vi "Preferences.vi"(7 "FileList":refnum<vi>, 11 "Files":T1[](array[typedef])) -> (0 "Settings out":T2={"Name of test"="", "Date"=timestamp(0 s since 1904-01-01), "Location"="", "Template"="", "Soundcard"="", "resolution"=32, "Sampling rate"=48000, "Ch1 Gain "=25.0, "Ch2 Gain"=10.0, "Sample time (s)"=0.3, "Pre-trigger (s)"=0.01, "Hammer Threshold"=10.0, "Positions"=12, "Taps/Position"=5, "Set Names"="", "Freq resolution"=10.0, "Hammer cutoff"=0.0, "Mic cutoff"=0.0, "Double bounce "=0.0, "Hammer Cal"=10.0, "dB Offset"=0.0, "Accel Cal"=10.0, "Vibrometer Cal"=0.0, "Mic Cal"=0.0, "Output"=2, "Voltage Cal"=0.01, "Vibrometer Port"="ASRL27::INSTR", "Range"=4, "High Pass"=2, "Bandwidth"=4, "X Range"=[], "Y Range"=[], "dB Spread"=0.0, "Trigger"=0, "Ch_1"=25, "Ch_2"=25, "flip?"=FALSE, "60Hz"=FALSE, "Time offset"=0.0, "Piezo Cal"=1.0, "Default Notes"="", "Tom"=FALSE} {"Ch_2" min=1 step=1; "Ch_1" min=1 max=100 step=1; "Trigger" items=["Hammer (force)", "Self-tap", "Spacebar"]; "Bandwidth" items=["1 kHz"=1, "5 kHz"=5, "10 kHz"=10, "25 kHz"=25, "50 kHz"=50, "100 kHz"=100]; "High Pass" items=["Off", "13 Hz", "104 Hz"]; "Range" items=["10 mm/s"=1, "20 mm/s"=2, "50 mm/s"=5, "100 mm/s"=10, "200 mm/s"=20, "500 mm/s"=50, "1 m/s"=100, "2 m/s"=200]; "Output" items=["Accelerometer", "Speed (from acceleration)", "Microphone", "Vibrometer", "Piezo"]; "Voltage Cal" format="%#_13g"; "Ch2 Gain" format="%#_13g"; "Ch1 Gain" format="%#_13g"; "Double bounce" min=0.0; "Mic cutoff" min=0.0 format="%#_4g"; "Hammer cutoff" min=0.0 format="%#_4g"; "Freq resolution" min=0.0; "Pre-trigger (s)" format="%#_13g"; "Date" format="%<%H:%M\n%d/%m/%y>T"; "resolution" items=["16 bit"=16, "24 bit"=24, "32 bit"=32]; "Sampling rate" items=["22050 samp/s"=22050, "44100 samp/s"=44100, "48000 samp/s"=48000]}, 1 "Success?":bool, 3 "Fixed Files":T1[](array[typedef]))   [LabVIEW 2022 SP3]
uses:
  PreferencesControl.ctl
  Curtin1_Label.ctl
  Mic/Mic_Global.vi
panel:
  out "Cover":bool
  in  "Tab Control":T3(tab)
  in  "CSV?":bool=TRUE
  in  "DAQ":bool
  in  "Vibrometer":bool
  in  "View":bool
  in  "Device":u16(ring) items=["485B39 200083408035100798118210422", "MacBook Pro Microphone", "Microsoft Teams Audio"]
  out "Data Folder:":path=path "/Users/crogers/Desktop/Curtin2/Data"
  in  "Data Folder":bool
  out "Path to preferences":path
  out "Current ScratchPad Settings":string
  in  "Trigger":u16(ring) items=["Hammer (force)", "Self-tap"]
  in  "60Hz?":bool
  in  "F<0?":bool
  in  "Add Color":bool
  in  "Viewing":T4={"Alerts"=FALSE, "Log X Axis"=TRUE, "dB scale"=TRUE, "Averaging"=TRUE, "Fade"=0.8181818181818182, "Centroids?"=TRUE, "line thickness"=1} {"Fade" scale=0.0..1.0}
  in  "Plot Colors":u16(ring) items=["Last Saved", "24 Colors", "rear"]
  in  "Note Files":u16(ring) items=["Default Notes", "Laser Notes", "Original Notes", "Testing Notes"]
  in  "Default Notes":string
  in  "Save As":bool
  in  "remove csv":bool
  in  "Reset":bool
  in  "Type":bool
  in  "Name":string(combo)
  in  "Selection":T5(radio)
  in  "open Folder":bool
  in  "Cancel Button":bool
  in  "OK Button":bool
  out "Version":string
  # "Hz"
  # "dB"
  # "dB"
  # "sec"
  # "sec"
  # "mV/Pa"
  # "mV/m/s2"
  # "mV/mm/s"
  # "V/N"
  # "sec"
  # "sec"
  # "mV/N"
  # "a.u."
  # "a.u."
  # "sec"
  # "not visible"
  # "no fade"
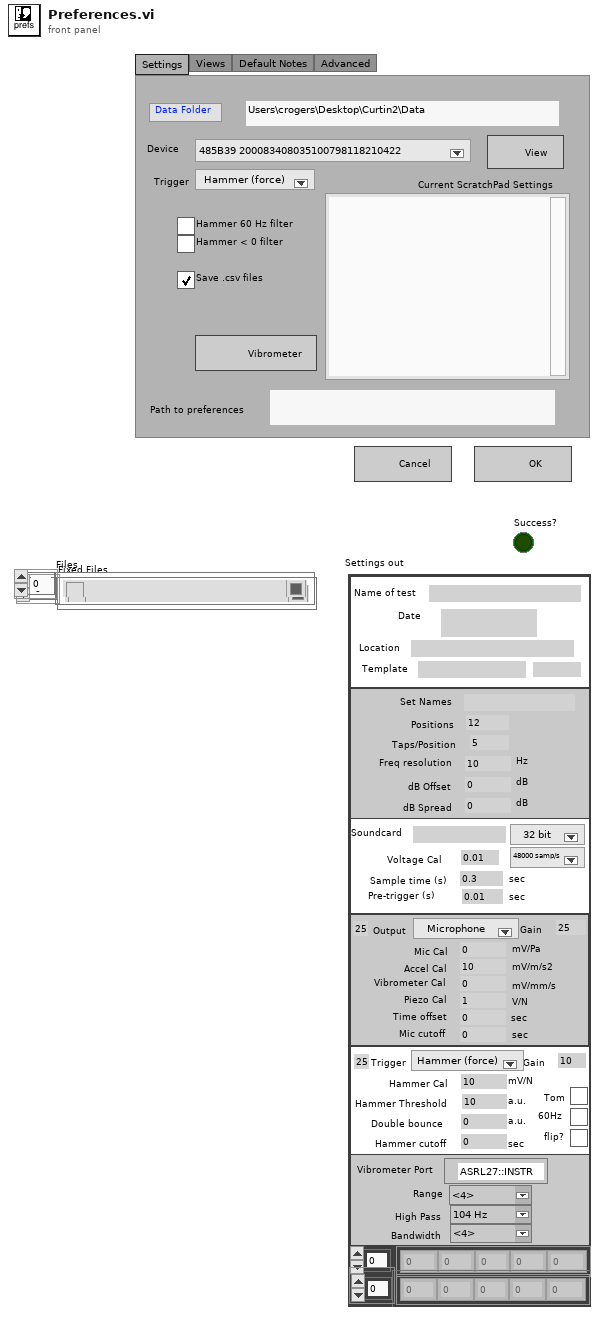
[diagram p1: front panel]
types:
  T1 = typedef "Curtin1_Label.ctl" = cluster{"Show?":bool, "Name":string, "Color":u32, "Path":path, "Show Notes":bool}
  T2 = typedef "PreferencesControl.ctl" = cluster{"Name of test":string, "Date":timestamp, "Location":string, "Template":string, "Soundcard":string, "resolution":u16, "Sampling rate":u16, "Ch1 Gain ":dbl, "Ch2 Gain":dbl, "Sample time (s)":dbl, "Pre-trigger (s)":dbl, "Hammer Threshold":dbl, "Positions":i16, "Taps/Position":i16, "Set Names":string, "Freq resolution":dbl, "Hammer cutoff":dbl, "Mic cutoff":dbl, "Double bounce ":dbl, "Hammer Cal":dbl, "dB Offset":dbl, "Accel Cal":dbl, "Vibrometer Cal":dbl, "Mic Cal":dbl, "Output":u16, "Voltage Cal":dbl, "Vibrometer Port":refnum<visa-resource-name>, "Range":u16, "High Pass":u16, "Bandwidth":u16, "X Range":cluster{"Minimum":dbl, "Maximum":dbl, "Increment":dbl, "Minor Increment":dbl, "Start":dbl}[], "Y Range":cluster{"Minimum":dbl, "Maximum":dbl, "Increment":dbl, "Minor Increment":dbl, "Start":dbl}[], "dB Spread":dbl, "Trigger":u16, "Ch_1":u8, "Ch_2":u8, "flip?":bool, "60Hz":bool, "Time offset":dbl, "Piezo Cal":dbl, "Default Notes":string, "Tom":bool}
  T3 = enum32{"Settings", "Views", "Default Notes", "Advanced"}
  T4 = cluster{"Alerts":bool, "Log X Axis":bool, "dB scale":bool, "Averaging":bool, "Fade":dbl, "Centroids?":bool, "line thickness":u8}
  T5 = enum32{"No Selection", "Rename", "Recalculate", "Export", "Delete", "Duplicate"}
  T6 = enum32{"Invalid", "Default", "Floating", "Floating/Auto-Hide", "Modal"}
  T7 = enum16{"big-endian, network order", "native, host order", "little-endian"}
  T8 = enum32{"No Selection", "Rename", "Recalculate", "Export", "Delete"}
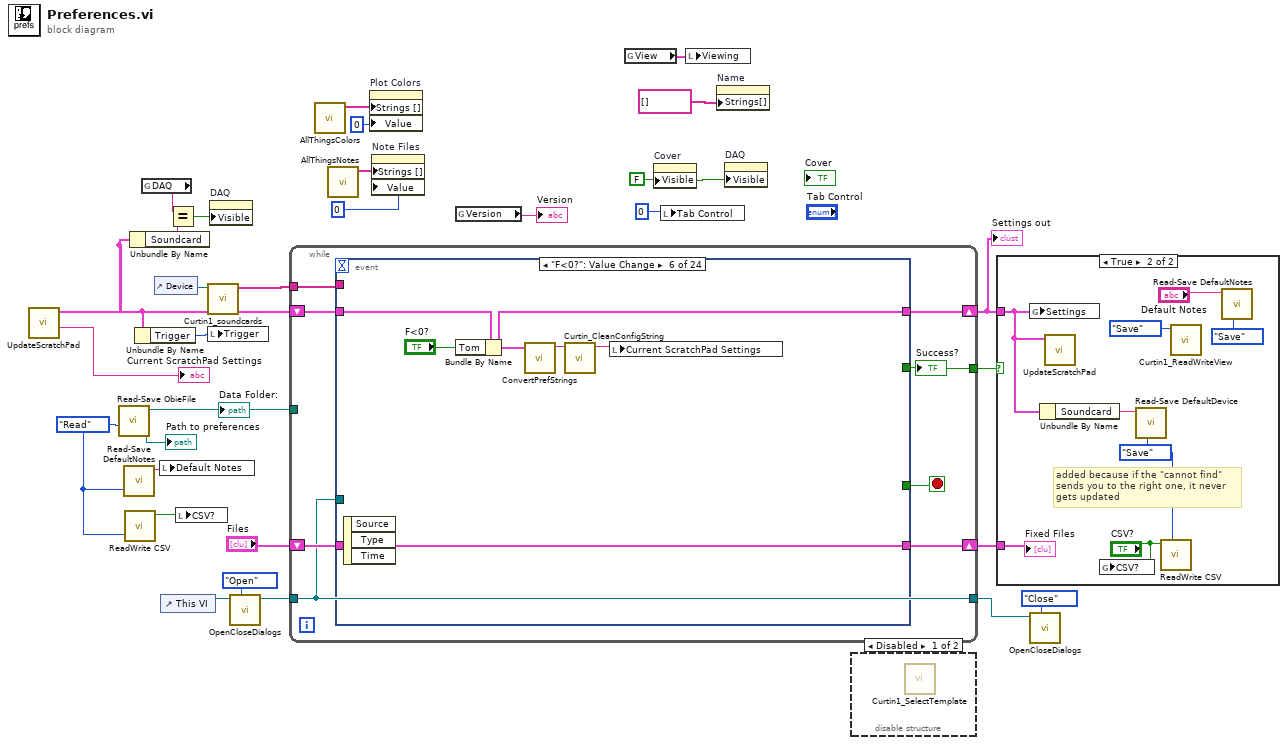
[diagram p0: block diagram]
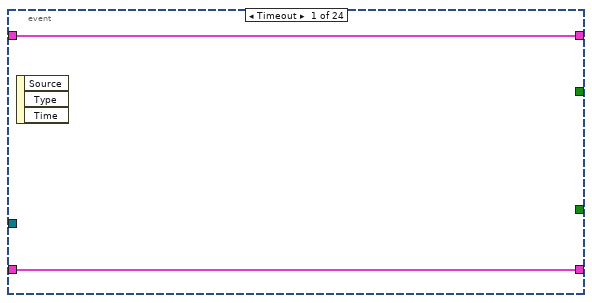
[diagram p4: hidden frame]
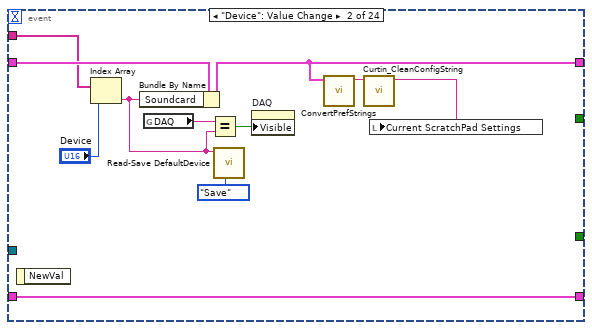
[diagram p5: hidden frame]
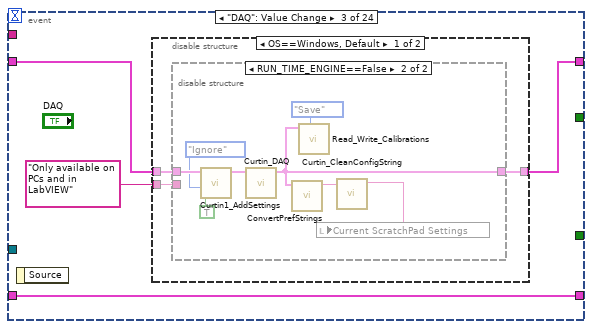
[diagram p6: hidden frame]
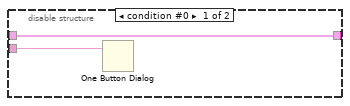
[diagram p7: hidden frame]
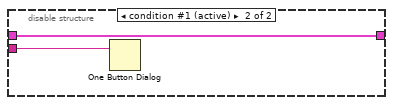
[diagram p8: hidden frame]
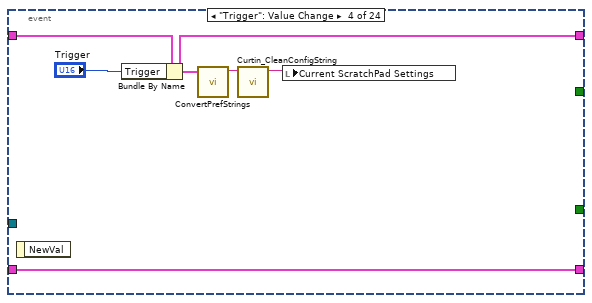
[diagram p9: hidden frame]
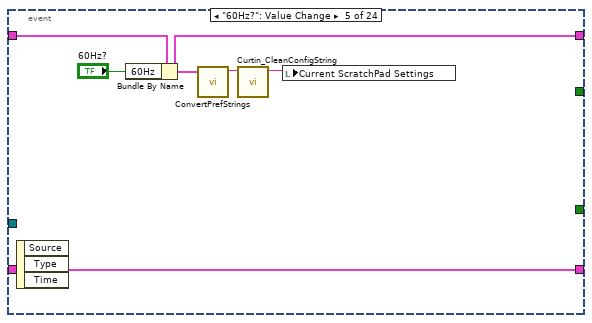
[diagram p10: hidden frame]
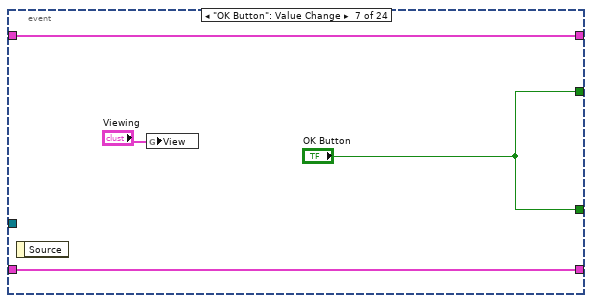
[diagram p11: hidden frame]
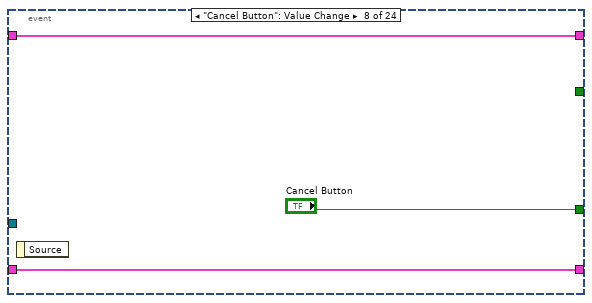
[diagram p12: hidden frame]
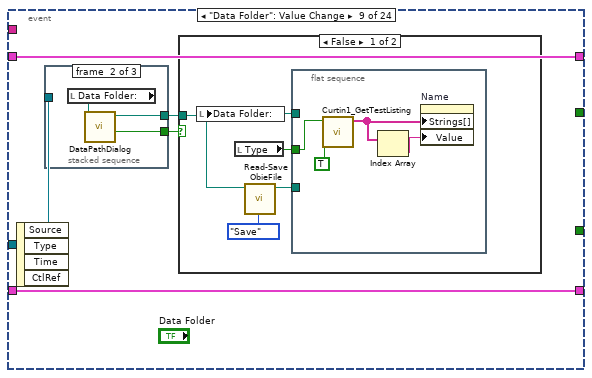
[diagram p13: hidden frame]
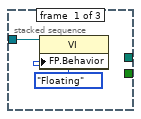
[diagram p14: hidden frame]
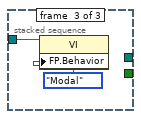
[diagram p15: hidden frame]
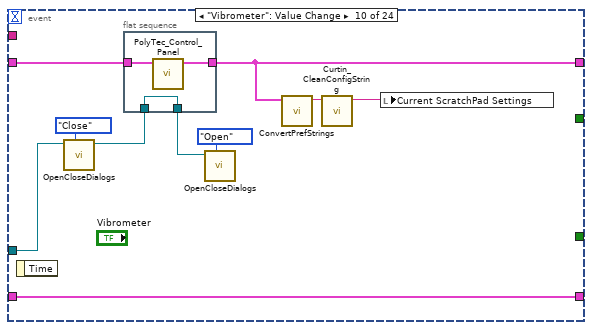
[diagram p17: hidden frame]
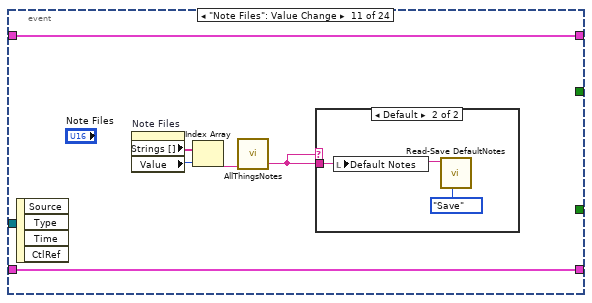
[diagram p18: hidden frame]
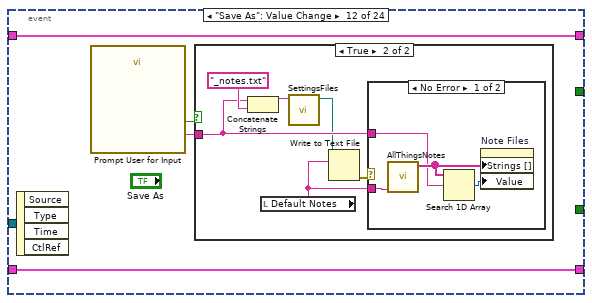
[diagram p20: hidden frame]
diagram:
  w10 = FALSE ("Visible")
  w2 = enum16{"Save", "Read"}."Read" ("Task")
  n1 = call "UpdateScratchPad.vi"() -> ("Settings"=→"Current ScratchPad Settings":string, "Settings Out"=w9:T2)  [unwired: 10 in]
  n2 = call "Read-Save ObieFile.vi"("Task"=w2) -> ("Pref Path"=→"Path to preferences":path, "DataPath Out"=w25:path)  [unwired: 8 in, 1 out]
  "Data Folder:" <- w25
  n3 = call "Read-Save DefaultNotes.vi"("Task"=w2) -> ("Notes Out"=w29:string)  [unwired: 9 in, 1 out]
  n4 = call "ReadWrite CSV.vi"("Task"=w2) -> ("csv Out"=w1:bool)  [unwired: 10 in]
  n5 = Unbundle By Name(w9) -> ("Soundcard"=w12:string)
  n6 = Unbundle By Name(w9) -> ("Trigger"=w20:u16)
  n7 = global read "Mic_Global.vi" "DAQ"() -> (w11:string)
  n8 = control-ref of="Device"() -> (w24:refnum<vi>)
  n9 = local write "Default Notes"(w29) -> ()
  n10 = control-ref of="This VI"() -> (w6:refnum<vi>)
  n11 = Equal?(x=w11, y=w12) -> (x = y?=w13:bool)
  n12 = local write "CSV?"(w1) -> ()
  n13 = call "Curtin1_soundcards.vi"("Settings In"=w9, "device:"=w24) -> ("Settings Out"=w19:T2, "Devices"=w26:string[])  [unwired: 8 in]
  n14 = local write "Trigger"(w20) -> ()
  n15 = property on="DAQ" class="Bool"("Visible"=w13) -> ()  [unwired: 2 in, 2 out]
  n16 = call "OpenCloseDialogs.vi"("Task"=enum16{"Open", "Close"}."Open", "VI in"=w6) -> ("VI out"=w3:refnum<vi>)  [unwired: 8 in, 1 out]
  n17 = while {
    tunnel: w26 -> [w39]
    shift-right: [w37] -> w30
    shift-left: w19 -> [w38]
    tunnel: [w36] -> w28
    tunnel: w25 -> [_]
    shift-right: [w35] -> w16
    shift-left: "Files" -> [w34]
    tunnel: [w33] -> w4
    tunnel: w3 -> [w33]
    stop <- w40 stop-if-true
    n18 = event shown="[5] \"F<0?\": Value Change" {
      selector: _ -> [_ _ _ _ _ _ _ _ _ _ _ _ _ _ _ _ _ _ _ _ _ _ _ _]
      dyn-events: _ -> [_ _ _ _ _ _ _ _ _ _ _ _ _ _ _ _ _ _ _ _ _ _ _ _]
      timeout: _ -> [_ _ _ _ _ _ _ _ _ _ _ _ _ _ _ _ _ _ _ _ _ _ _ _]
      tunnel: [_ _ _ _ _ _ "OK Button" "Cancel Button" _ _ _ _ _ _ _ _ _ _ _ _ _ _ _ w252] -> w40
      tunnel: w39 -> [_ w51 _ _ _ _ _ _ _ _ _ _ _ _ _ _ _ _ _ _ _ _ _ _]
      tunnel: [_ _ _ _ _ _ "OK Button" _ _ _ _ _ _ _ _ _ _ _ _ _ _ _ _ _] -> w36
      tunnel: w38 -> [w42 w52 w54 w78 w84 w90 w93 w96 w102 w126 w136 w142 w154 w161 w172 w177 w187 w193 w195 w204 w218 w228 w248 w251]
      tunnel: [w42 w44 w55 w74 w81 w87 w93 w96 w102 w124 w136 w142 w154 w161 w172 w177 w187 w193 w195 w202 w218 w228 w248 w251] -> w37
      tunnel: [w41 w50 w57 w76 w83 w89 w91 w95 w100 w127 w131 w139 w153 w155 w171 w176 w185 w192 w194 w203 w217 w227 w249 w250] -> w35
      tunnel: w34 -> [w41 w50 w57 w76 w83 w89 w91 w95 w100 w127 w131 w139 w153 w155 w171 w176 w185 w192 w194 w203 _ w227 w249 w250]
      tunnel: w33 -> [_ _ _ _ _ _ _ _ w98 w121 _ _ _ _ _ _ _ _ _ w200 _ w224 _ _]
      event Timeout {
        n19 = event-data() -> ()  [unwired: 1 in, 3 out]
      }
      event "Device": Value Change {
        n20 = event-data() -> ()  [unwired: 1 in, 1 out]
        n21 = Index Array(array=w51, index="Device") -> (element=w46:string)
        n22 = Bundle By Name(cluster=w52, "Soundcard"=w46) -> (w44:T2)
        n23 = global read "Mic_Global.vi" "DAQ"() -> (w48:string)
        n24 = Equal?(x=w48, y=w46) -> (x = y?=w47:bool)
        n25 = call "Read-Save DefaultDevice.vi"("Task"=enum16{"Save", "Read"}."Save", "Soundcard"=w46) -> ()  [unwired: 8 in, 2 out]
        n26 = property on="DAQ" class="Bool"("Visible"=w47) -> ()  [unwired: 2 in, 2 out]
        n27 = call "ConvertPrefStrings.vi"("Settings"=w44) -> ("String Out"=w45:string)  [unwired: 9 in, 1 out]
        n28 = call "Curtin_CleanConfigString.vi"("String in"=w45) -> ("String out"=w43:string)  [unwired: 10 in]
        n29 = local write "Current ScratchPad Settings"(w43) -> ()
      }
      event "DAQ": Value Change {
        n30 = event-data() -> ()  [unwired: 1 in, 1 out]
        n31 = disable-structure shown="OS==Windows, Default" {
          disable-tunnel: "Only available on PCs and in LabVIEW" ("message") -> [w60 w72]
          disable-tunnel: w54 -> [w59 w71]
          disable-tunnel: [w58 w71] -> w55
          frame condition #0 {
            n32 = disable-structure shown="RUN_TIME_ENGINE==False" {
              disable-tunnel: w60 -> [w62 _]
              disable-tunnel: w59 -> [w61 w70]
              disable-tunnel: [w61 w68] -> w58
              frame condition #0 {
                n33 = One Button Dialog(message=w62) -> ()  [unwired: 1 in, 1 out]
              }
              frame condition #1 (active) {
                n34 = call "Curtin1_AddSettings.vi"("Date?"=TRUE, "Check?"=enum16{"Ignore", "Check", "Replace"}."Ignore", "Settings in"=w70) -> ("Settings Out"=w69:T2)  [unwired: 7 in, 1 out]
                n35 = call "Curtin_DAQ.vi"("Settings"=w69) -> ("Settings out"=w68:T2)  [unwired: 10 in]
                n36 = call "ConvertPrefStrings.vi"("Settings"=w68) -> ("String Out"=w66:string)  [unwired: 9 in, 1 out]
                n37 = call "Read_Write_Calibrations.vi"("Task"=enum16{"Save", "Read", "List"}."Save", "Settings in"=w68) -> ()  [unwired: 7 in, 3 out]
                n38 = call "Curtin_CleanConfigString.vi"("String in"=w66) -> ("String out"=w65:string)  [unwired: 10 in]
                n39 = local write "Current ScratchPad Settings"(w65) -> ()
              }
            }
          }
          frame condition #1 (active) {
            n40 = One Button Dialog(message=w72) -> ()  [unwired: 1 in, 1 out]
          }
        }
      }
      event "Trigger": Value Change {
        n41 = event-data() -> ()  [unwired: 1 in, 1 out]
        n42 = Bundle By Name(cluster=w78, "Trigger"="Trigger") -> (w74:T2)
        n43 = call "ConvertPrefStrings.vi"("Settings"=w74) -> ("String Out"=w75:string)  [unwired: 9 in, 1 out]
        n44 = call "Curtin_CleanConfigString.vi"("String in"=w75) -> ("String out"=w73:string)  [unwired: 10 in]
        n45 = local write "Current ScratchPad Settings"(w73) -> ()
      }
      event "60Hz?": Value Change {
        n46 = event-data() -> ()  [unwired: 1 in, 3 out]
        n47 = Bundle By Name(cluster=w84, "60Hz"="60Hz?") -> (w81:T2)
        n48 = call "ConvertPrefStrings.vi"("Settings"=w81) -> ("String Out"=w82:string)  [unwired: 9 in, 1 out]
        n49 = call "Curtin_CleanConfigString.vi"("String in"=w82) -> ("String out"=w80:string)  [unwired: 10 in]
        n50 = local write "Current ScratchPad Settings"(w80) -> ()
      }
      event "F<0?": Value Change {
        n51 = event-data() -> ()  [unwired: 1 in, 3 out]
        n52 = Bundle By Name(cluster=w90, "Tom"="F<0?") -> (w87:T2)
        n53 = call "ConvertPrefStrings.vi"("Settings"=w87) -> ("String Out"=w88:string)  [unwired: 9 in, 1 out]
        n54 = call "Curtin_CleanConfigString.vi"("String in"=w88) -> ("String out"=w86:string)  [unwired: 10 in]
        n55 = local write "Current ScratchPad Settings"(w86) -> ()
      }
      event "OK Button": Value Change {
        n56 = event-data() -> ()  [unwired: 1 in, 1 out]
        n57 = global write "Mic_Global.vi" "View"("Viewing") -> ()
      }
      event "Cancel Button": Value Change {
        n58 = event-data() -> ()  [unwired: 1 in, 1 out]
      }
      event "Data Folder": Value Change {
        n59 = event-data() -> ()  [unwired: 1 in, 4 out]
        n60 = stacked-sequence {
          tunnel: [_ w106 _] -> w101
          tunnel: [_ w105 _] -> w99
          tunnel: w98 -> [w104 _ w109]
          frame #0 {
            n61 = property class="VI"(reference=w104, "FP.Behavior"=T6."Floating" ("Front Panel Window:Behavior")) -> ()  [unwired: 1 in, 2 out]
          }
          frame #1 {
            n62 = local read "Data Folder:"() -> (w107:path)
            n63 = call "DataPathDialog.vi"("Path"=w107) -> ("canceled?"=w105:bool, "Path out"=w106:path)  [unwired: 9 in]
          }
          frame #2 {
            n64 = property class="VI"(reference=w109, "FP.Behavior"=T6."Modal" ("Front Panel Window:Behavior")) -> ()  [unwired: 1 in, 2 out]
          }
        }
        n65 = case shown="False" w99 {
          tunnel: w101 -> [w111 _]
          frame False {
            n66 = local write "Data Folder:"(w111) -> ()
            n67 = local read "Type"() -> (w113:bool)
            n68 = call "Read-Save ObieFile.vi"("Task"=enum16{"Save", "Read"}."Save", "DataPath"=w111) -> ("DataPath Out"=w110:path)  [unwired: 7 in, 2 out]
            n69 = flat-sequence {
              tunnel: w111 -> [_]
              tunnel: w113 -> [w115]
              tunnel: w110 -> [_]
              frame #0 {
                n70 = call "Curtin1_GetTestListing.vi"("Rebuild"=TRUE, "Type"=w115) -> ("Array"=w117:string[])  [unwired: 9 in]
                n71 = Index Array(array=w117) -> (element=w116:string)  [unwired: 1 in]
                n72 = property on="Name" class="CmbBox"("Strings[]"=w117, "Value"=w116) -> ()  [unwired: 2 in, 2 out]
              }
            }
          }
          frame True {
          }
        }
      }
      event "Vibrometer": Value Change {
        n73 = event-data() -> ()  [unwired: 1 in, 1 out]
        n74 = call "OpenCloseDialogs.vi"("Task"=enum16{"Open", "Close"}."Close", "VI in"=w121) -> ("VI out"=w119:refnum<vi>)  [unwired: 8 in, 1 out]
        n75 = flat-sequence {
          tunnel: w126 -> [w130]
          tunnel: [w129] -> w124
          tunnel: [w128] -> w120
          tunnel: w119 -> [w128]
          frame #0 {
            n76 = call "PolyTec_Control_Panel.vi"("Settings in"=w130) -> ("Settings Out"=w129:T2)  [unwired: 8 in, 2 out]
          }
        }
        n77 = call "OpenCloseDialogs.vi"("Task"=enum16{"Open", "Close"}."Open", "VI in"=w120) -> ()  [unwired: 8 in, 2 out]
        n78 = call "ConvertPrefStrings.vi"("Settings"=w124) -> ("String Out"=w125:string)  [unwired: 9 in, 1 out]
        n79 = call "Curtin_CleanConfigString.vi"("String in"=w125) -> ("String out"=w123:string)  [unwired: 10 in]
        n80 = local write "Current ScratchPad Settings"(w123) -> ()
      }
      event "Note Files": Value Change {
        n81 = event-data() -> ()  [unwired: 1 in, 4 out]
        n82 = property on="Note Files" class="Ring (strict)"() -> ("Strings []"=w135:string[], "Value"=w133:u16)  [unwired: 2 in, 2 out]
        n83 = Index Array(array=w135, index=w133) -> (element=w134:string)
        n84 = call "AllThingsNotes.vi"("Choice"=w134) -> ("Text"=w132:string)  [unwired: 9 in, 1 out]
        n85 = case shown="Default" w132 {
          tunnel: w132 -> [_ w137]
          frame "" {
          }
          frame Default {
            n86 = local write "Default Notes"(w137) -> ()
            n87 = call "Read-Save DefaultNotes.vi"("Task"=enum16{"Save", "Read"}."Save", "Notes"=w137) -> ()  [unwired: 8 in, 2 out]
          }
        }
      }
      event "Save As": Value Change {
        n88 = event-data() -> ()  [unwired: 1 in, 4 out]
        n89 = call "Prompt User for Input"() -> ("Filename"=w140:string, "OK"=w141:bool)  [unwired: 17 in, 1 out]
        n90 = case shown="True" w141 {
          tunnel: w140 -> [_ w146]
          frame False {
          }
          frame True {
            n91 = Concatenate Strings(w146, "_notes.txt" ("pattern")) -> (w145:string)
            n92 = local read "Default Notes"() -> (w147:string)
            n93 = call "SettingsFiles.vi"("settings file name"=w145) -> ("file path"=w144:path)  [unwired: 9 in, 1 out]
            n94 = Write to Text File(file (use dialog)=w144, text=w147) -> (error out=w143:errorcluster)  [unwired: 2 in, 2 out]
            n95 = case shown="No Error" w143 {
              tunnel: w147 -> [w152 _]
              tunnel: w146 -> [w149 _]
              frame No Error {
                n96 = call "AllThingsNotes.vi"("Choice"=w152) -> ("Array"=w150:string[])  [unwired: 9 in, 1 out]
                n97 = Search 1D Array(1D array=w150, element=w149) -> (index of element=w151:i32)  [unwired: 1 in]
                n98 = property on="Note Files" class="Ring (strict)"("Strings []"=w150, "Value"=w151) -> ()  [unwired: 2 in, 2 out]
              }
              frame Error {
              }
            }
          }
        }
      }
      event "Default Notes": Value Change {
        n99 = event-data() -> ()  [unwired: 1 in, 4 out]
      }
      event "Selection": Value Change {
        n100 = event-data() -> ()  [unwired: 1 in, 2 out]
        n101 = local read "Type"() -> (w156:bool)
        n102 = call "Curtin1_AdvancedPrefs.vi"("Type"=w156, "Selection"="Selection", "Instrument:Test Name"="Name") -> ("Selection out"=w158:T8, "message"=w157:string)  [unwired: 7 in]
        n103 = local write "Selection"(w158) -> ()
        n104 = case shown="Default" w157 {
          selector: w157 -> [_ w166]
          tunnel: w156 -> [_ w163]
          frame "" {
          }
          frame Default {
            n105 = One Button Dialog(message=w166) -> ()  [unwired: 1 in, 1 out]
            n106 = call "Curtin1_GetTestListing.vi"("Rebuild"=TRUE, "Type"=w163) -> ("Array"=w165:string[])  [unwired: 9 in]
            n107 = Index Array(array=w165) -> (element=w164:string)  [unwired: 1 in]
            n108 = property on="Name" class="CmbBox"("Strings[]"=w165, "Value"=w164) -> ()  [unwired: 2 in, 2 out]
          }
        }
      }
      event "Type": Value Change {
        n109 = event-data() -> ()  [unwired: 1 in, 2 out]
        n110 = property on="Cover" class="Bool (strict)"("Visible"=TRUE) -> ()  [unwired: 2 in, 2 out]
        n111 = call "Curtin1_GetTestListing.vi"("Rebuild"=FALSE, "Type"="Type") -> ("Array"=w175:string[])  [unwired: 9 in]
        n112 = Index Array(array=w175) -> (element=w174:string)  [unwired: 1 in]
        n113 = property on="Name" class="CmbBox"("Strings[]"=w175, "Value"=w174) -> (error out=w168:errorcluster)  [unwired: 2 in, 1 out]
        n114 = property on="Cover" class="Bool (strict)"(error in=w168, "Visible"=FALSE) -> ()  [unwired: 1 in, 2 out]
      }
      event "Tab Control": Value Change {
        n115 = event-data() -> ("NewVal"=w178:T3)  [unwired: 1 in]
        n116 = case shown="\"Advanced\"" w178 {
          frame "Settings", Default {
          }
          frame "Advanced" {
            n117 = property on="Name" class="CmbBox"() -> ("Strings[]"=w181:string[])  [unwired: 2 in, 2 out]
            n118 = Array Size(array=w181) -> (size(s)=w180:i32)
            n119 = case shown="0" w180 {
              tunnel: string[] ["Loading..."] ("Strings []") -> [_ w182]
              frame Default {
              }
              frame 0 {
                # "First Run"
                n120 = property on="Type" class="Bool (strict)"("Val(Sgnl)"=FALSE ("Value (Signaling)")) -> ()  [unwired: 2 in, 2 out]
                n121 = property on="Name" class="CmbBox"("Strings[]"=w182) -> ()  [unwired: 2 in, 2 out]
              }
            }
          }
        }
      }
      event "Reset": Value Change {
        n122 = event-data() -> ()  [unwired: 1 in, 1 out]
        n123 = call "Curtin1_GlobalFolder.vi"() -> ("LabVIEW Data Path"=w184:path)  [unwired: 1 in, 1 out]
        n124 = call "DefaultSettings.vi"("Task"=enum16{"Load to VI", "Save to Disk"}."Save to Disk", "path (use dialog)"=w184) -> ("No Errors?"=w186:bool)  [unwired: 9 in]
        n125 = case shown="False" w186 {
          frame False {
            n126 = One Button Dialog(message="Error in saving files") -> ()  [unwired: 1 in, 1 out]
          }
          frame True {
            n127 = One Button Dialog(message="Success") -> ()  [unwired: 1 in, 1 out]
          }
        }
      }
      event "open Folder": Value Change {
        n128 = event-data() -> ()  [unwired: 1 in, 1 out]
        n129 = call "Curtin1_GlobalFolder.vi"() -> ("LabVIEW Data Path"=w191:path)  [unwired: 1 in, 1 out]
        n130 = call "OpenFolder.vi"("LabVIEW Data Path"=w191) -> ()  [unwired: 11 in]
      }
      event "Name": Value Change {
        n131 = event-data() -> ()  [unwired: 1 in, 4 out]
      }
      event "View": Value Change {
        n132 = event-data() -> ()  [unwired: 1 in, 1 out]
        n133 = call "OpenCloseDialogs.vi"("Task"=enum16{"Open", "Close"}."Close", "VI in"=w200) -> ("error out"=w197:errorcluster, "VI out"=w196:refnum<vi>)  [unwired: 8 in]
        n134 = case shown="True" "View" {
          tunnel: w204 -> [w207 w214]
          tunnel: [w207 w209] -> w202
          tunnel: [w206 w208] -> w198
          tunnel: w197 -> [w206 w208]
          frame False {
          }
          frame True {
            n135 = call "Curtin1_AddSettings.vi"("Date?"=TRUE, "Check?"=enum16{"Ignore", "Check", "Replace"}."Ignore", "Settings in"=w214) -> ("Settings Out"=w215:T2)  [unwired: 7 in, 1 out]
            n136 = call "Curtin1_ViewMics.vi"("Settings"=w215) -> ("Settings Out"=w209:T2)  [unwired: 10 in]
            n137 = call "ConvertPrefStrings.vi"("Settings"=w209) -> ("String Out"=w213:string)  [unwired: 9 in, 1 out]
            n138 = call "Curtin_CleanConfigString.vi"("String in"=w213) -> ("String out"=w212:string)  [unwired: 10 in]
            n139 = local write "Current ScratchPad Settings"(w212) -> ()
          }
        }
        n140 = call "OpenCloseDialogs.vi"("Task"=enum16{"Open", "Close"}."Open", "error in (no error)"=w198, "VI in"=w196) -> ()  [unwired: 7 in, 2 out]
      }
      event "Plot Colors": Value Change {
        n141 = event-data() -> ()  [unwired: 1 in, 1 out]
        n142 = flat-sequence {
          tunnel: "FileList" -> [w223]
          tunnel: [w222] -> w217
          frame #0 {
            # "load into CurrentColors"
            n143 = property on="Plot Colors" class="Ring (strict)"() -> ("Strings []"=w220:string[], "Value"=w221:u16)  [unwired: 2 in, 2 out]
            n144 = Index Array(array=w220, index=w221) -> (element=w219:string)
            n145 = call "AllThingsColors.vi"("Choice"=w219) -> ()  [unwired: 10 in, 1 out]
          }
          frame #1 {
            # "replot"
            n146 = call "Recolor.vi"("Array in"=w223) -> ("Files"=w222:T1[])  [unwired: 10 in]
          }
        }
      }
      event "Add Color": Value Change {
        n147 = event-data() -> ()  [unwired: 1 in, 1 out]
        n148 = stacked-sequence {
          tunnel: [_ w232 _] -> w226
          tunnel: [_ w231 _] -> w225
          tunnel: w224 -> [w229 _ w233]
          frame #0 {
            n149 = property class="VI"(reference=w229, "FP.Behavior"=T6."Floating" ("Front Panel Window:Behavior")) -> ()  [unwired: 1 in, 2 out]
          }
          frame #1 {
            n150 = call "Curtin_SaveColor.vi"() -> ("New Color"=w232:string, "Good?"=w231:bool)  [unwired: 10 in]
          }
          frame #2 {
            n151 = property class="VI"(reference=w233, "FP.Behavior"=T6."Modal" ("Front Panel Window:Behavior")) -> ()  [unwired: 1 in, 2 out]
          }
        }
        n152 = case shown="True" w225 {
          tunnel: w227 -> [_ w242]
          tunnel: w226 -> [_ w237]
          frame False {
          }
          frame True {
            # "Save color file"
            n153 = for {
              tunnel: w242 -> [w247] mode=indexing
              tunnel: [w246] -> w239 mode=indexing
              n154 = Unbundle By Name(w247) -> ("Color"=w246:u32)
            }
            n155 = call "GetColorFilePath.vi"("String"=w237) -> ("name"=w235:string, "path"=w236:path)  [unwired: 9 in]
            n156 = Write to Binary File(file (use dialog)=w236, data=w239, 5:FALSE ("prepend array or string size? (T)"), 9:T7."big-endian, network order" ("byte order (0:big-endian, network order)")) -> (error out=w238:errorcluster)  [unwired: 2 in, 2 out]
            n157 = case shown="No Error" w238 {
              tunnel: w235 -> [w244 _]
              frame No Error {
                n158 = call "AllThingsColors.vi"() -> ("Possible Colors"=w245:string[])  [unwired: 11 in]
                n159 = Search 1D Array(1D array=w245, element=w244) -> (index of element=w243:i32)  [unwired: 1 in]
                n160 = property on="Plot Colors" class="Ring (strict)"("Strings []"=w245, "Value"=w243) -> ()  [unwired: 2 in, 2 out]
              }
              frame Error {
              }
            }
          }
        }
      }
      event "remove csv": Value Change {
        n161 = event-data() -> ()  [unwired: 1 in, 1 out]
        n162 = call "Delete csv.vi"() -> ()  [unwired: 12 in]
      }
      event Panel Close? {
        w252 = TRUE ("Discard?")
        n163 = event-data() -> ()  [unwired: 1 in, 4 out]
        n164 = event-data("Discard?"=w252) -> ()  [unwired: 1 in, 1 out]
      }
    }
    "Success?" <- w36
  }
  "Settings out" <- w30
  n165 = call "AllThingsColors.vi"() -> ("Possible Colors"=w15:string[])  [unwired: 11 in]
  n166 = call "AllThingsNotes.vi"() -> ("Array"=w23:string[])  [unwired: 10 in, 1 out]
  n167 = property on="Plot Colors" class="Ring (strict)"("Strings []"=w15, "Value"=0) -> ()  [unwired: 2 in, 2 out]
  n168 = property on="Note Files" class="Ring (strict)"("Strings []"=w23, "Value"=0) -> ()  [unwired: 2 in, 2 out]
  n169 = global read "Mic_Global.vi" "Version"() -> (→"Version":string)
  n170 = global read "Mic_Global.vi" "View"() -> (w21:T4)
  n171 = property on="Cover" class="Bool (strict)"("Visible"=w10) -> ()  [unwired: 2 in, 2 out]
  n172 = local write "Tab Control"(0) -> ()
  n173 = local write "Viewing"(w21) -> ()
  n174 = property on="Name" class="CmbBox"("Strings[]"=string[] [] ("Strings []")) -> ()  [unwired: 2 in, 2 out]
  n175 = property on="DAQ" class="Bool"("Visible"=w10) -> ()  [unwired: 2 in, 2 out]
  n176 = disable-structure shown="Disabled" {
    frame Disabled {
      n177 = call "Curtin1_SelectTemplate.vi"() -> ()  [unwired: 10 in, 2 out]
    }
    frame Enabled {
    }
  }
  n178 = case shown="True" w28 {
    tunnel: w30 -> [_ w256]
    tunnel: w16 -> [_ w257]
    frame False {
    }
    frame True {
      w254 = enum16{"Save", "Read"}."Save" ("Task")
      # "added because if the \"cannot find\"\nsends you to the right one, it never\ngets updated"
      n179 = global write "Mic_Global.vi" "Settings"(w256) -> ()
      n180 = Unbundle By Name(w256) -> ("Soundcard"=w255:string)
      n181 = call "UpdateScratchPad.vi"("Settings"=w256) -> ()  [unwired: 9 in, 2 out]
      n182 = global write "Mic_Global.vi" "CSV?"("CSV?") -> ()
      n183 = call "Read-Save DefaultDevice.vi"("Task"=w254, "Soundcard"=w255) -> ()  [unwired: 8 in, 2 out]
      n184 = call "ReadWrite CSV.vi"("Task"=w254, "csv?"="CSV?") -> ()  [unwired: 9 in, 1 out]
      n185 = call "Curtin1_ReadWriteView.vi"("Task"=enum16{"Read", "Save"}."Save") -> ()  [unwired: 8 in, 3 out]
      n186 = call "Read-Save DefaultNotes.vi"("Task"=enum16{"Save", "Read"}."Save", "Notes"="Default Notes") -> ()  [unwired: 8 in, 2 out]
      "Fixed Files" <- w257
    }
  }
  n187 = call "OpenCloseDialogs.vi"("Task"=enum16{"Open", "Close"}."Close", "VI in"=w4) -> ()  [unwired: 8 in, 2 out]
